vi "Get Max No. of pull-ins.vi"(8 "error in (no error)":errorcluster, 11 "Motor in":refnum<class "Motor.lvclass">) -> (0 "error out":errorcluster, 2 "Max No. of pull-ins":u8=5, 3 "Motor out":refnum<class "Motor.lvclass">)   [LabVIEW 2016, in "Hardware.lvlib" / "Motor.lvlib" / "Motor.lvclass"]
doc: "get max No. of pull-ins by considering the setting of SW closed loop\nreturn 0 no matter what, if SW closed loop is false"
uses:
  <userlib>/Common Components/Hardware/Motor/Motor/Motor.lvclass
  <userlib>/Common Components/Hardware/Motor/Motor/Motor.lvclass/Motor.ctl
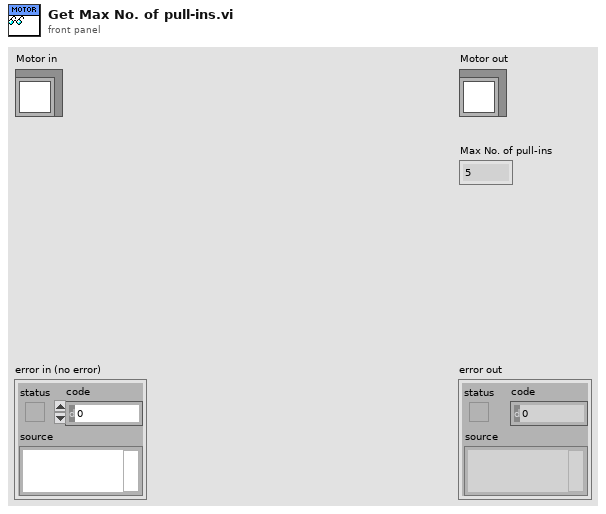
[diagram p1: front panel]
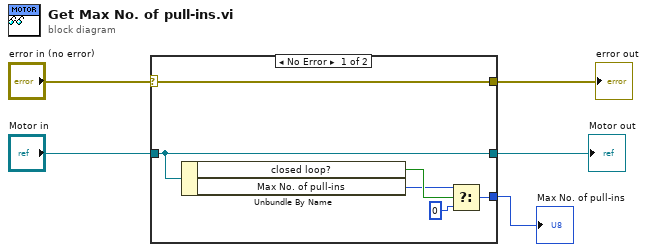
[diagram p0: block diagram]
diagram:
  n1 = case shown="No Error" "error in (no error)" {
    selector: "error in (no error)" -> [w11 w12]
    tunnel: [w11 w12] -> w4
    tunnel: [w10 w13] -> w2
    tunnel: "Motor in" -> [w10 w13]
    tunnel: [w8 _] -> w1
    frame No Error {
      n2 = Unbundle By Name(w10) -> ("closed loop?"=w9:bool, "Max No. of pull-ins"=w7:u8)
      n3 = Select(t=w7, s=w9, f=u8 0) -> (s? t:f=w8:u8)
    }
    frame Error {
    }
  }
  "error out" <- w4
  "Motor out" <- w2
  "Max No. of pull-ins" <- w1
